vi "Correct Data.vi"(8 "error in":errorcluster, 10 "Data In":refnum<class "Data.lvclass">, 11 "Alicat Device in":refnum<class "Alicat Device.lvclass">) -> (0 "error out":errorcluster, 2 "Data Out":refnum<class "Data.lvclass">, 3 "Alicat Device out":refnum<class "Alicat Device.lvclass">)   [LabVIEW 2014, in "Alicat Lib.lvlib" / "Alicat Device.lvclass"]
uses:
  Alicat Device.lvclass
  reusable/Data/Data.lvclass
  Data/Alicat Data.lvclass
  Configurable Device/Configurable Device.lvclass/Configurable Device.ctl
  Data/Alicat Data.lvclass/Alicat Data.ctl
  Alicat Device.lvclass/Alicat Device.ctl
  Data/Accessors/Write Data.vi
  Data/Accessors/Read Data.vi
  Data/Accessors/Read ID.vi
  Configurable Device/Accessors/Read Cal Equation.vi
  Configurable Device/Accessors/Read Model.vi
  <vilib>/gmath/NI_Gmath.lvlib
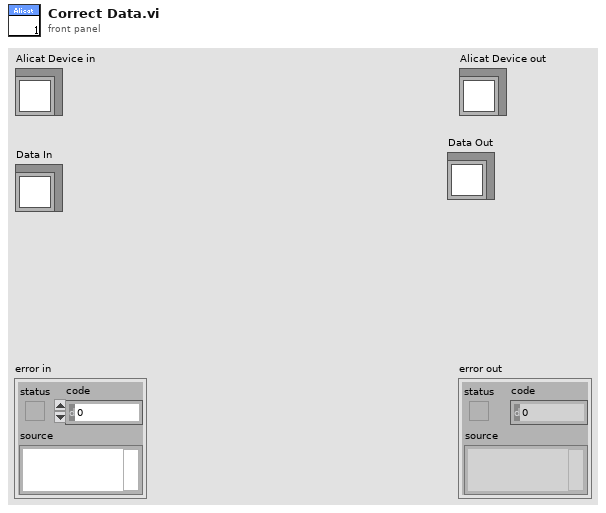
[diagram p1: front panel]
types:
  T1 = cluster{"P":sgl, "T":sgl, "Q":sgl, "Qsp":sgl, "Q0":sgl}
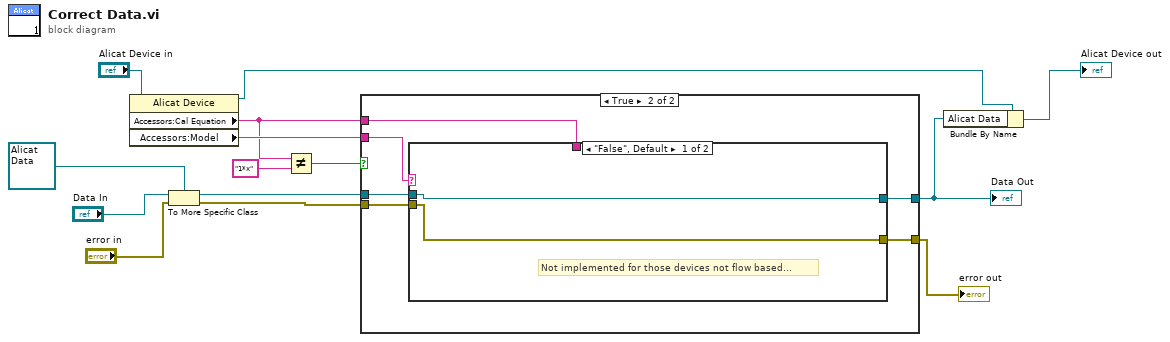
[diagram p0: block diagram]
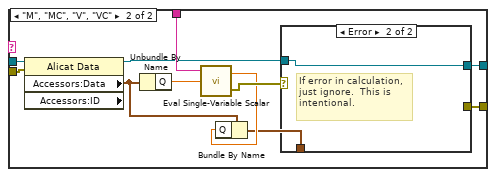
[diagram p3: hidden frame]
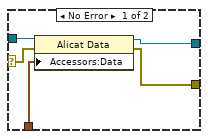
[diagram p4: hidden frame]
diagram:
  n1 = property class="Alicat Device"(reference="Alicat Device in") -> (reference out=w3:refnum<class "Alicat Device.lvclass">, "Accessors:Cal Equation"=w7:string, "Accessors:Model"=w10:string)  [unwired: 1 in, 1 out]
  n2 = To More Specific Class(target class=refnum<class "Alicat Data.lvclass"> refnum ("Alicat Lib.lvlib:Alicat Data"), reference="Data In", error in="error in") -> (specific class reference=w9:refnum<class "Alicat Data.lvclass">, error out=w8:errorcluster)
  n3 = Not Equal?(x=w7, y="1*x") -> (x != y?=w5:bool)
  n4 = case shown="True" w5 {
    tunnel: w10 -> [_ w22]
    tunnel: w9 -> [w15 w21]
    tunnel: w8 -> [w16 w20]
    tunnel: w7 -> [_ w19]
    tunnel: [w15 w18] -> w1
    tunnel: [w16 w17] -> w4
    frame False {
    }
    frame True {
      n5 = case shown="\"False\", Default" w22 {
        tunnel: w21 -> [w24 w35]
        tunnel: w20 -> [w23 w34]
        tunnel: w19 -> [_ w33]
        tunnel: [w24 w26] -> w18
        tunnel: [w23 w25] -> w17
        frame "False", Default {
          # "Not implemented for those devices not flow based..."
        }
        frame "M", "MC", "V", "VC" {
          n6 = property class="Alicat Data" props=["Accessors:Data", "Accessors:ID"](reference=w35, error in=w34) -> (reference out=w31:refnum<class "Alicat Data.lvclass">, "Accessors:Data"=w30:T1)  [unwired: 2 out]
          n7 = Unbundle By Name(w30) -> ("Q"=w32:sgl)
          n8 = call <vilib>:"Eval Single-Variable Scalar.vi"("x value"=w32, "formula"=w33) -> ("error out"=w29:errorcluster, "y value"=w28:dbl)  [unwired: 1 in]
          n9 = Bundle By Name(cluster=w30, "Q"=w28) -> (w27:T1)
          n10 = case shown="Error" w29 {
            selector: w29 -> [w36 _]
            tunnel: w31 -> [w40 w41]
            tunnel: w27 -> [w39 _]
            tunnel: [w38 w41] -> w26
            tunnel: [w37 _] -> w25
            frame No Error {
              n11 = property class="Alicat Data"(reference=w40, error in=w36, "Accessors:Data"=w39) -> (reference out=w38:refnum<class "Alicat Data.lvclass">, error out=w37:errorcluster)
            }
            frame Error {
              # "If error in calculation, \njust ignore.  This is intentional."
            }
          }
        }
      }
    }
  }
  "error out" <- w4
  "Data Out" <- w1
  n12 = Bundle By Name(cluster=w3, "Alicat Data"=w1) -> (→"Alicat Device out":refnum<class "Alicat Device.lvclass">)
